vi "C867_DLL_Test.vi"(8 "error in":errorcluster caption="entrée d'erreur") -> (0 "error out":errorcluster caption="sortie d'erreur")   [LabVIEW 2026]
uses:
  Controls/TypeDef_FGV.ctl
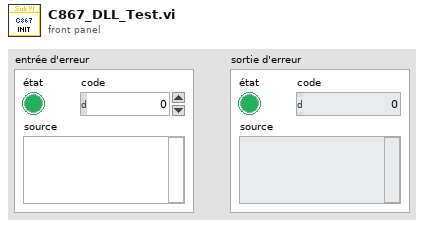
[diagram p1: front panel]
types:
  T1 = typedef "TypeDef_FGV.ctl" = enum16{"Initialize", "Write", "Read"}
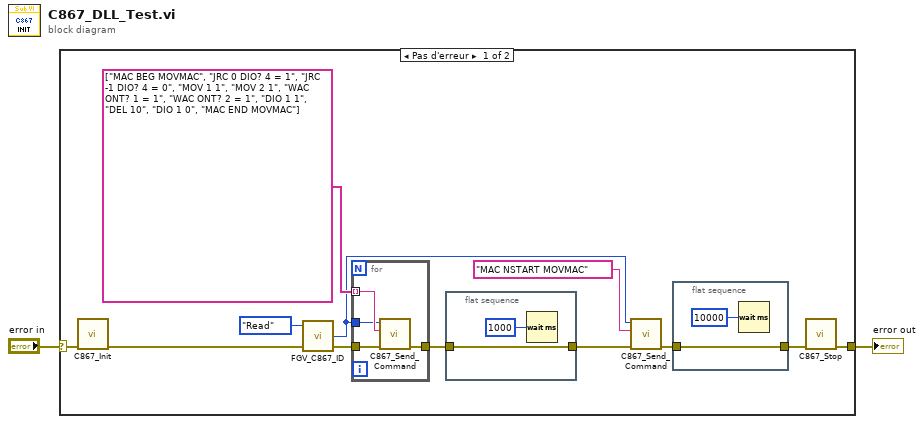
[diagram p0: block diagram]
diagram:
  n1 = case shown="Pas d'erreur" "error in" {
    selector: "error in" -> [w12 w23]
    tunnel: [w13 w23] -> w1
    frame No Error {
      n2 = call "C867_Init.vi"("error in"=w12) -> ("error out"=w10:errorcluster)  [unwired: 10 in]
      n3 = call "FGV_C867_ID.vi"("error in"=w10, "Action"=TypeDef_FGV."Read") -> ("error out"=w9:errorcluster, "ID"=w7:i32)  [unwired: 2 in]
      n4 = for {
        tunnel: string[] ["MAC BEG MOVMAC", "JRC 0 DIO? 4 = 1", "JRC -1 DIO? 4 = 0", "MOV 1 1", "MOV 2 1", "WAC ONT? 1 = 1", "WAC ONT? 2 = 1", "DIO 1 1", "DEL 10", "DIO 1 0", "MAC END MOVMAC"] -> [w22] mode=indexing
        tunnel: w7 -> [w21]
        tunnel: w9 -> [w20]
        tunnel: [w19] -> w8
        n5 = call "C867_Send_Command.vi"("entrée d'erreur (pas d'erreur)"=w20, "szCommand"=w22, "ID en entrée"=w21) -> ("sortie d'erreur"=w19:errorcluster)  [unwired: 6 in, 2 out]
      }
      n6 = flat-sequence {
        tunnel: [w17] -> w6
        tunnel: w8 -> [w17]
        frame #0 {
          n7 = Wait (ms)(milliseconds to wait=u32 1000 ("attente (ms)")) -> ()  [unwired: 1 out]
        }
      }
      n8 = call "C867_Send_Command.vi"("entrée d'erreur (pas d'erreur)"=w6, "szCommand"="MAC NSTART MOVMAC", "ID en entrée"=w7) -> ("sortie d'erreur"=w4:errorcluster)  [unwired: 6 in, 2 out]
      n9 = flat-sequence {
        tunnel: [w15] -> w3
        tunnel: w4 -> [w15]
        frame #0 {
          n10 = Wait (ms)(milliseconds to wait=u32 10000 ("attente (ms)")) -> ()  [unwired: 1 out]
        }
      }
      n11 = call "C867_Stop.vi"("error in"=w3) -> ("error out"=w13:errorcluster)  [unwired: 10 in]
    }
    frame Error {
    }
  }
  "error out" <- w1
